vi "SetSpec.vi"(8 "error in (no error)":errorcluster, 10 "Spec":string, 11 "reference in":refnum<class "TestView_Tree_Single.lvclass">) -> (0 "error out":errorcluster, 3 "reference in":refnum<class "TestView_Tree_Single.lvclass">)   [LabVIEW 2022 SP3, in "TestView_Tree_Single.lvlib" / "TestView_Tree_Single.lvclass"]
uses:
  TestView_Tree_Single.lvclass
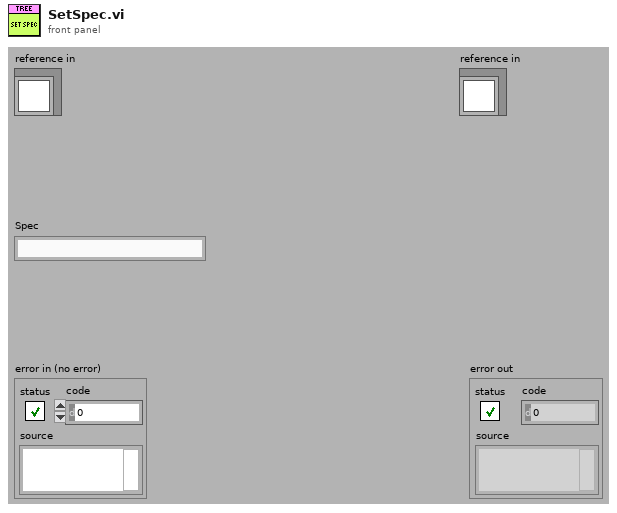
[diagram p1: front panel]
types:
  T1 = typedef "TestView_Tree_Single.lvlib/TestView_Tree_Single.lvclass/ObjectAttributes.ctl" = cluster{"Front Panel":refnum<vi>, "Last_Item":string, "Config":T2, "Title":string, "User":string, "TreeRef":refnum<vi>, "Active DUT":i32, "Status":T3, "SN":string, "Spec":string}
  T2 = typedef "TestView_Tree_Single.lvlib/TestView_Tree_Single.lvclass/Config.ctl" = cluster{"default":string}
  T3 = typedef "TestView_Base.lvlibp/TestView_Base.lvclass/ViewStatus.ctl" = enum16{"Testing", "Ready", "Logout", "Login", "PASS", "FAIL", "FAULT", "ABORTED"}
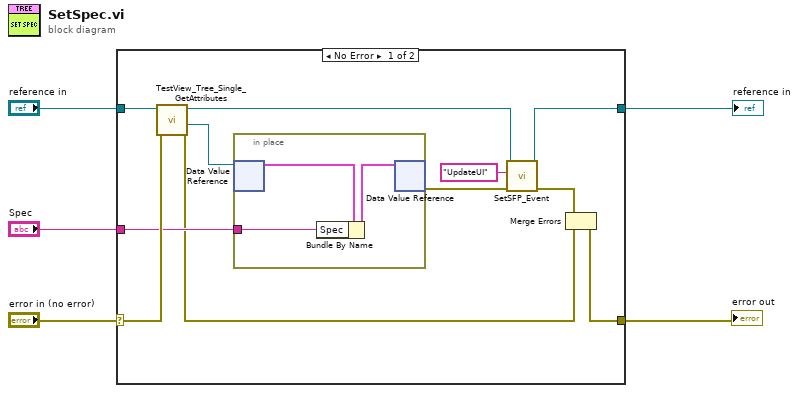
[diagram p0: block diagram]
diagram:
  n1 = case shown="No Error" "error in (no error)" {
    selector: "error in (no error)" -> [w16 w21]
    tunnel: [w9 w21] -> w4
    tunnel: [w7 w20] -> w2
    tunnel: "reference in" -> [w15 w20]
    tunnel: "Spec" -> [w13 _]
    frame No Error {
      n2 = call "TestView_Tree_Single_GetAttributes.vi"("error in (no error)"=w16, "reference in"=w15) -> ("error out"=w10:errorcluster, "DataRef"=w14:refnum<data-value>, "reference out"=w8:refnum<class "TestView_Tree_Single.lvclass">)  [unwired: 6 in, 1 out]
      n3 = in-place {
        in-place-border: w13 -> [w17]
        n4 = in-place-dvr #1(w14) -> (w19:T1)  [unwired: 1 out]
        n5 = Bundle By Name(cluster=w19, "Spec"=w17) -> (w18:T1)
        n6 = in-place-dvr #1(w18) -> (w12:errorcluster)  [unwired: 1 out]
      }
      n7 = call-dynamic "SetSFP_Event.vi"("error in (no error)"=w12, "msg"="UpdateUI", "reference in"=w8) -> ("error out"=w11:errorcluster, "reference out"=w7:refnum<class "TestView_Tree_Single.lvclass">)  [unwired: 7 in]
      n8 = Merge Errors(w11, w10) -> (w9:errorcluster)
    }
    frame Error {
    }
  }
  "error out" <- w4
  "reference in" <- w2
